vi "Anti_deadband_PVG.vi"(1 "x":sgl) -> (0 "y":sgl)   [LabVIEW 2017]
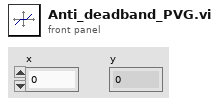
[diagram p1: front panel]
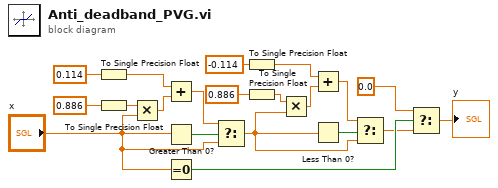
[diagram p0: block diagram]
diagram:
  n1 = To Single Precision Float(number=0.114 ("t")) -> (single precision float=w7:sgl)
  n2 = To Single Precision Float(number=0.886 ("t")) -> (single precision float=w17:sgl)
  n3 = Multiply(x=w17, y="x") -> (x*y=w20:sgl)
  n4 = Add(x=w7, y=w20) -> (x+y=w2:sgl)
  n5 = Greater Than 0?(x="x") -> (x > 0?=w1:bool)
  n6 = Equal To 0?(x="x") -> (x = 0?=w12:bool)
  n7 = Select(t=w2, s=w1, f="x") -> (s? t:f=w15:sgl)
  n8 = To Single Precision Float(number=-0.114 ("t")) -> (single precision float=w9:sgl)
  n9 = To Single Precision Float(number=0.886 ("t")) -> (single precision float=w19:sgl)
  n10 = Multiply(x=w19, y=w15) -> (x*y=w4:sgl)
  n11 = Add(x=w9, y=w4) -> (x+y=w3:sgl)
  n12 = Less Than 0?(x=w15) -> (x < 0?=w5:bool)
  n13 = Select(t=w3, s=w5, f=w15) -> (s? t:f=w10:sgl)
  n14 = Select(t=sgl 0.0, s=w12, f=w10) -> (s? t:f=→"y":sgl)
